vi "spectrum.vi"(11 "Array":u32[][](array[numeric])) -> (3 "XY Graph":cluster{i32[], u32[]}(graph))   [LabVIEW 2014]
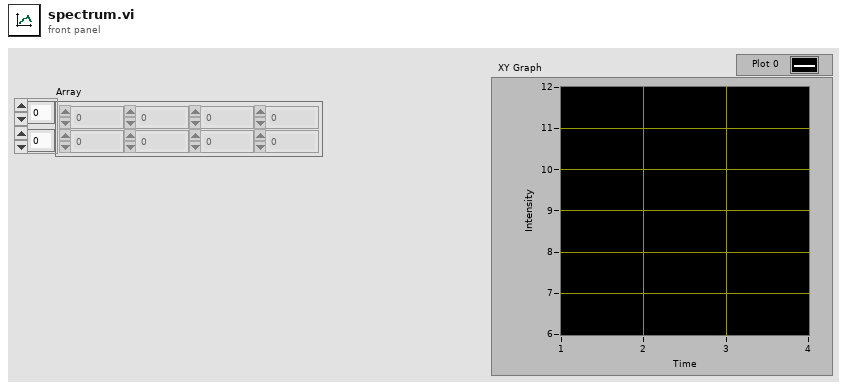
[diagram p1: front panel]
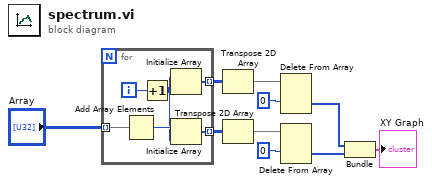
[diagram p0: block diagram]
diagram:
  n1 = for {
    tunnel: "Array" -> [w16] mode=indexing
    tunnel: [w15] -> w10 mode=indexing
    tunnel: [w11] -> w7 mode=indexing
    i -> [w13]
    n2 = Add Array Elements(numeric array=w16) -> (sum=w14:u32)
    n3 = Increment(x=w13) -> (x+1=w12:i32)
    n4 = Initialize Array(w12, w12) -> (w11:i32[])
    n5 = Initialize Array(w14, w12) -> (w15:u32[])
  }
  n6 = Transpose 2D Array(2D array=w7) -> (transposed array=w6:i32[][])
  n7 = Transpose 2D Array(2D array=w10) -> (transposed array=w9:u32[][])
  n8 = Delete From Array(array=w6, index (row)=0 ("index")) -> (deleted portion=w1:i32[])  [unwired: 2 in, 1 out]
  n9 = Delete From Array(array=w9, index (row)=0 ("index")) -> (deleted portion=w4:u32[])  [unwired: 2 in, 1 out]
  n10 = Bundle(w1, w4) -> (→"XY Graph":cluster{i32[], u32[]})  [unwired: 1 in]
